vi "errorHandler.vi"(7 "pid":string, 8 "error in":errorcluster, 9 "language":i32, 10 "errNbr":i32, 11 "connection ID":refnum<k5>) -> (0 "error out 2":errorcluster, 3 "connection ID out":refnum<k5>)   [LabVIEW 2016, in "amc_api.lvlib"]
uses:
  amc_api.lvlib
panel:
  out "jsonRespIn":string
  out "JSON-response":string="{\"jsonrpc\":\"2.0\",\"method\":\"\",\"params\":[5,1.245,true,\"name\"],\"id\":\"1\"}"
  out "JSON request":string
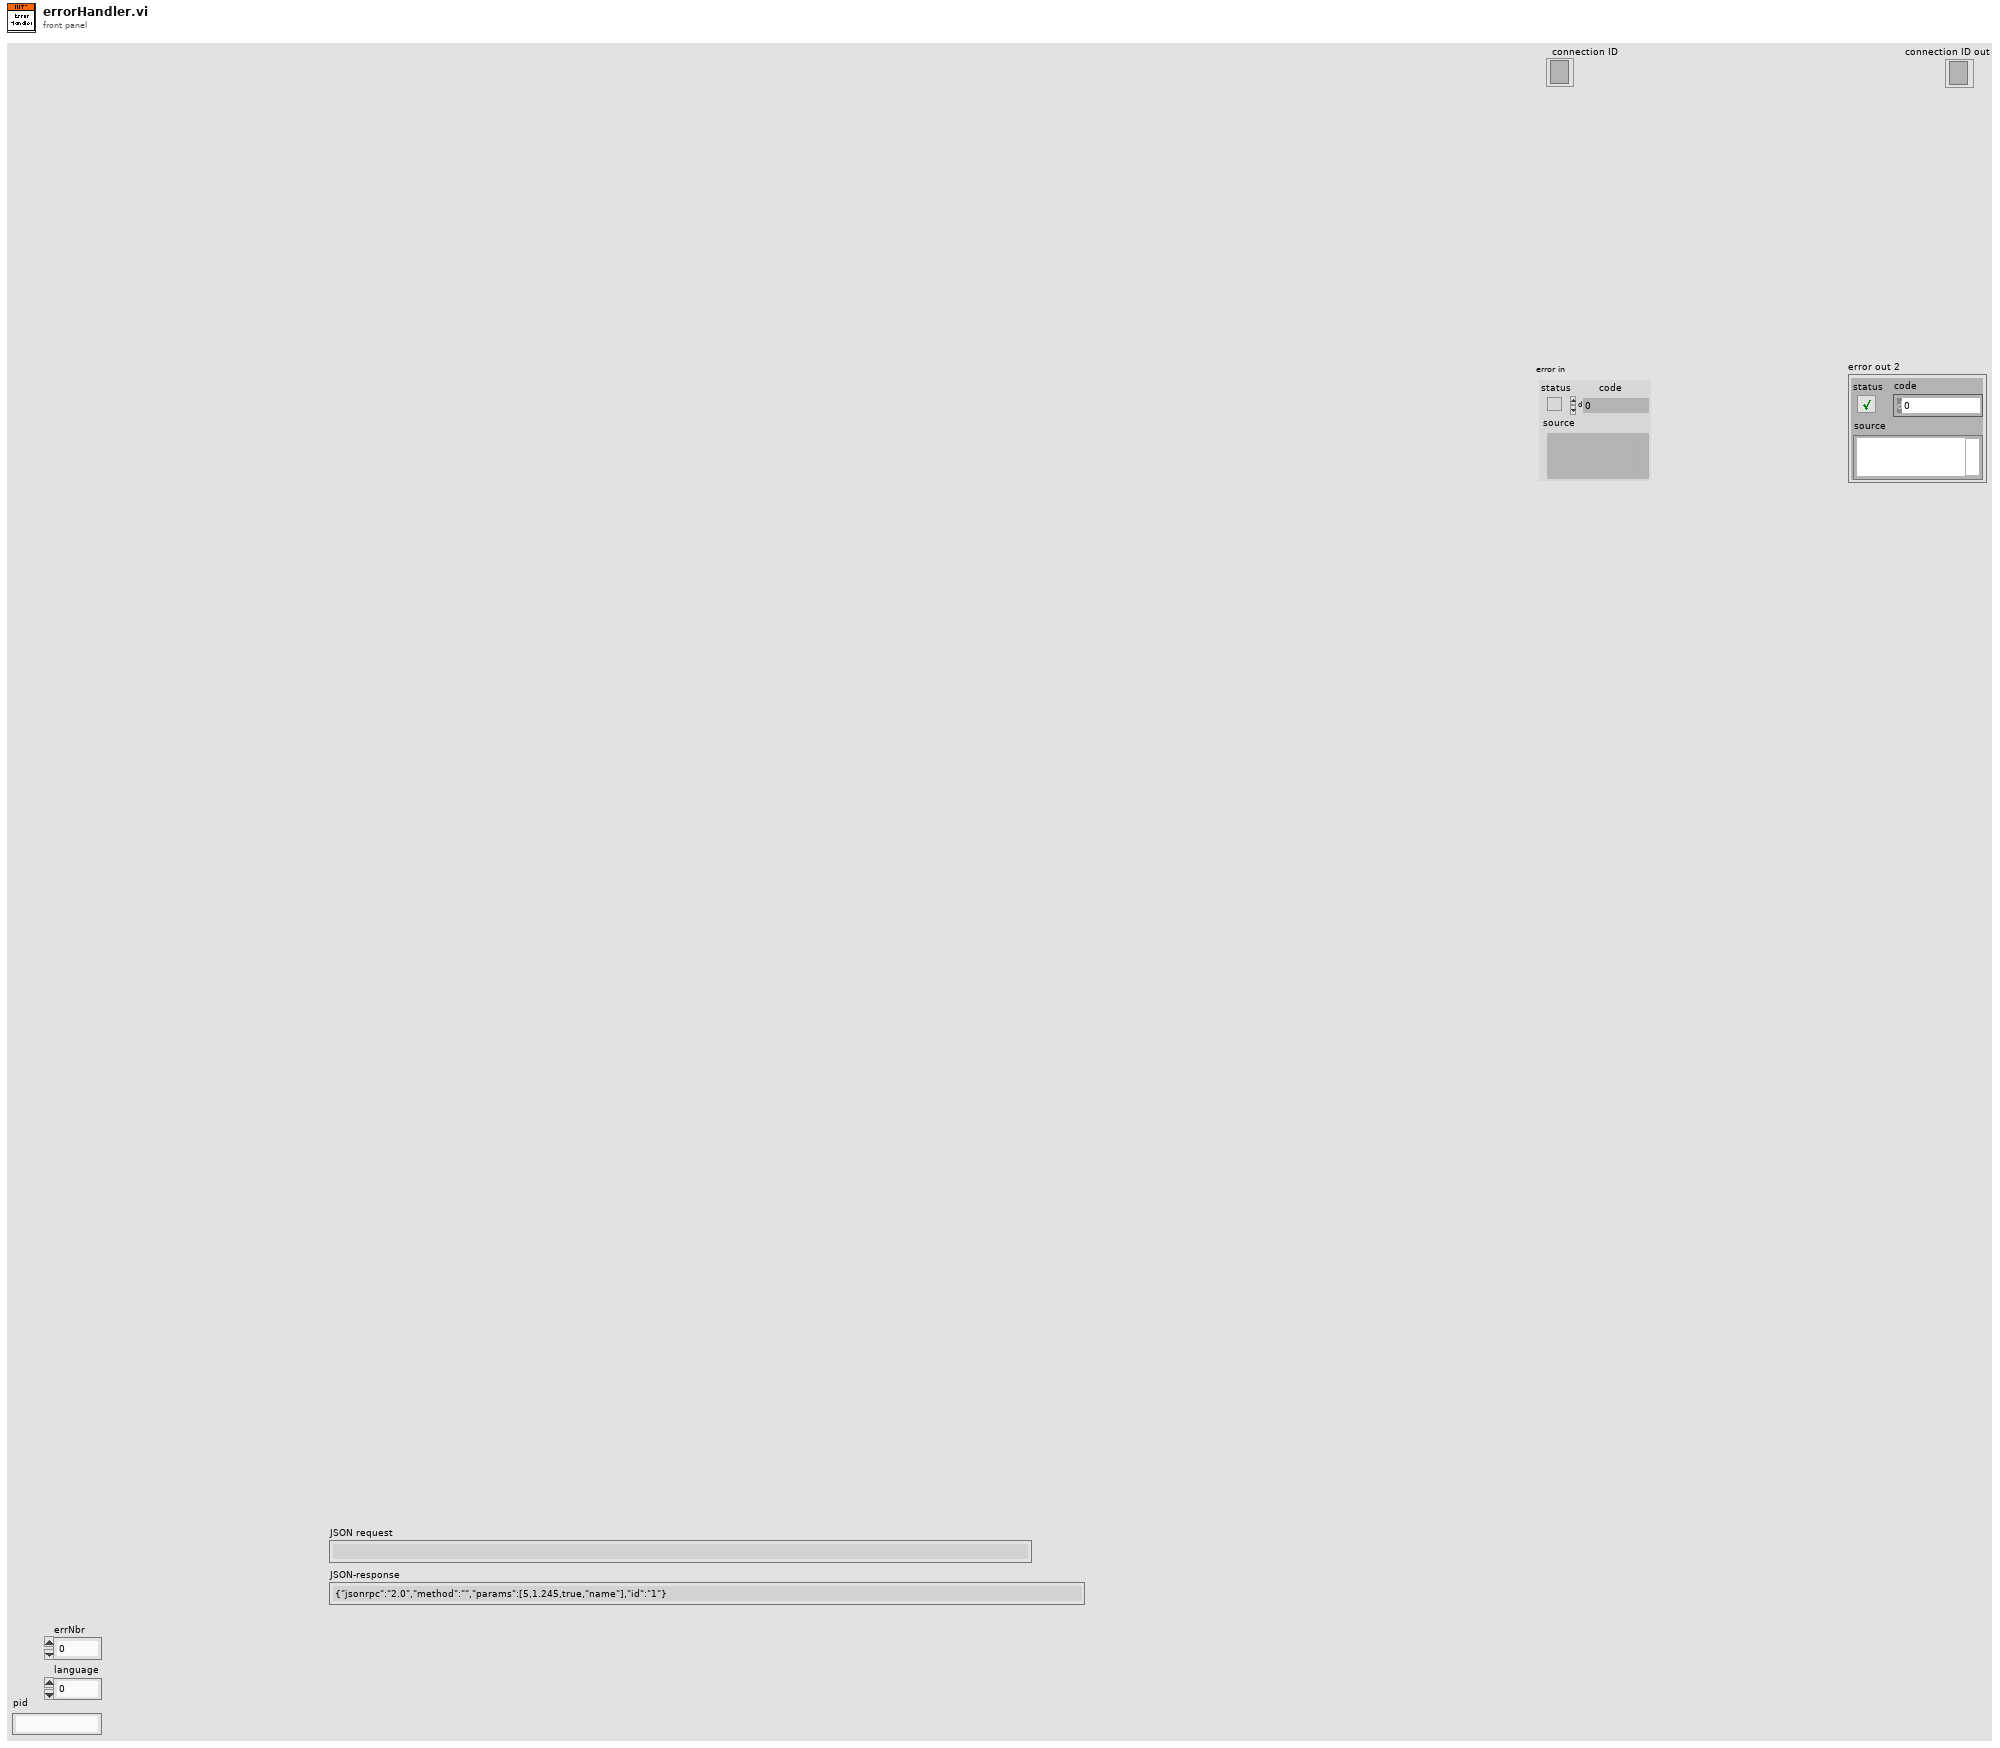
[diagram p1: front panel]
types:
  T1 = cluster{"jsonrpc":string, "method":string, "params":string[], "id":string, "api":i32, "pid":string}
  T2 = enum16{"Standard", "Buffered", "CRLF", "Immediate"}
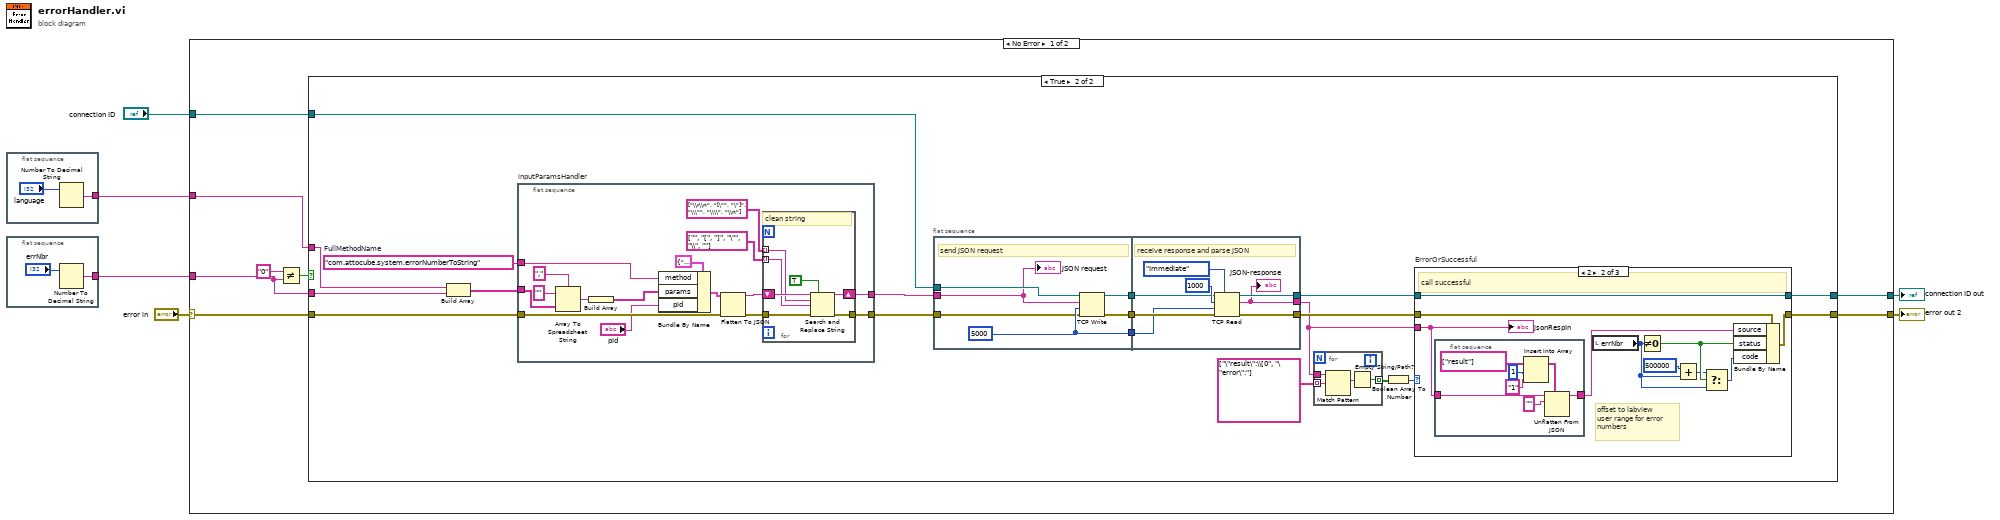
[diagram p0: block diagram]
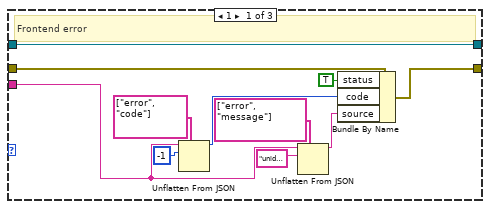
[diagram p3: hidden frame]
diagram:
  n1 = flat-sequence "in_integer" {
    tunnel: [w7] -> w2
    frame #0 {
      n2 = Number To Decimal String(number="language") -> (decimal integer string=w7:string)  [unwired: 1 in]
    }
  }
  n3 = flat-sequence "in_integer" {
    tunnel: [w9] -> w1
    frame #0 {
      n4 = Number To Decimal String(number="errNbr") -> (decimal integer string=w9:string)  [unwired: 1 in]
    }
  }
  n5 = case shown="No Error" "error in" {
    selector: "error in" -> [w14 w112]
    tunnel: [w18 w112] -> w6
    tunnel: [w17 w111] -> w5
    tunnel: "connection ID" -> [w16 w111]
    tunnel: w2 -> [w13 _]
    tunnel: w1 -> [w12 _]
    frame No Error {
      n6 = Not Equal?(x="0", y=w12) -> (x != y?=w15:bool)
      n7 = case shown="True" w15 {
        tunnel: [w20 w30] -> w18
        tunnel: [w19 w29] -> w17
        tunnel: w16 -> [w19 w28]
        tunnel: w12 -> [_ w23]
        tunnel: w14 -> [w20 w24]
        tunnel: w13 -> [_ w22]
        frame False {
        }
        frame True {
          w25 = "com.attocube.system.errorNumberToString"  # FullMethodName
          n8 = Build Array ("ParametersArrayString")(w22, w23) -> (w21:string[])
          n9 = flat-sequence "inputParamsHandler" {
            tunnel: [w43] -> w27
            tunnel: w21 -> [w50]
            tunnel: w24 -> [w48]
            tunnel: [w45] -> w26
            tunnel: w25 -> [w51]
            frame #0 {
              n10 = Array To Spreadsheet String(delimiter (Tab)=",", array=w50, 3:"" ("format string")) -> (spreadsheet string=w53:string)
              n11 = Build Array "Build Array"(w53) -> (w49:string[])
              n12 = Bundle By Name(cluster=T1 {"jsonrpc"="2.0", "method"="com.attocube.amc.res.setRESReadOutFreq", "params"=[], "id"="1", "api"=2, "pid"=""}, "method"=w51, "params"=w49, "pid"="pid") -> (w52:T1)
              n13 = Flatten To JSON(anything=w52, error in (no error)=w48) -> (JSON string=w44:string, 11:w46:errorcluster)  [unwired: 1 in]
              n14 = for {
                tunnel: string[] ["\\r\\n", "[\"", "\"]", "\\\"", "\\\\", "\\n"] ("search string") -> [w59] mode=indexing
                tunnel: string[] ["", "[", "]", "\"", "\\", ""] ("replace string (\"\")") -> [w58] mode=indexing
                shift-right: [w61] -> w43
                shift-left: w44 -> [w60]
                tunnel: w46 -> [w57]
                tunnel: [w56] -> w45
                # "clean string"
                n15 = Search and Replace String(replace all?=TRUE ("replace all? (F)"), input string=w60, search string=w59, replace string=w58, error in=w57) -> (result string=w61:string, error out=w56:errorcluster)  [unwired: 3 in, 2 out]
              }
            }
          }
          n16 = flat-sequence {
            tunnel: w28 -> [w102]
            tunnel: [w100] -> w39
            tunnel: [w101] -> w38
            tunnel: w26 -> [w97]
            tunnel: [w99] -> w37
            tunnel: w27 -> [w98]
            tunnel: [w106] -> w33
            tunnel: w39 -> [w108]
            tunnel: w38 -> [w107]
            tunnel: [w104] -> w32
            tunnel: w37 -> [w105]
            tunnel: [w103] -> w31
            frame #0 {
              w99 = 5000 ("timeout ms (25000)")
              # "send JSON request"
              n17 = TCP Write(connection ID=w102, data in=w98, error in (no error)=w97, 9:w99) -> (connection ID out=w100:refnum<k5>, error out=w101:errorcluster)  [unwired: 1 out]
              "JSON request" <- w98
            }
            frame #1 {
              # "receive response and parse JSON"
              n18 = TCP Read(connection ID=w108, bytes to read=1000, error in (no error)=w107, 7:T2."Immediate" ("mode (standard)"), 9:w105) -> (connection ID out=w106:refnum<k5>, data out=w103:string, error out=w104:errorcluster)
              "JSON-response" <- w103
            }
          }
          n19 = for {
            tunnel: string[] ["\"result\":\\[0", "\"error\":"] ("path") -> [w65] mode=indexing
            tunnel: [w63] -> w35 mode=indexing
            tunnel: w31 -> [w66]
            n20 = Match Pattern(string=w66, regular expression=w65) -> (match substring=w64:string)  [unwired: 1 in, 3 out]
            n21 = Empty String/Path?(string/path=w64) -> (empty?=w63:bool)
          }
          n22 = Boolean Array To Number(Boolean array=w35) -> (number=w34:u32)
          n23 = case "ErrorOrSuccessful" shown="2" w34 {
            tunnel: w31 -> [w69 w84 _]
            tunnel: w33 -> [w70 w87 w96]
            tunnel: [w70 w87 w96] -> w29
            tunnel: [w71 w85 w95] -> w30
            tunnel: w32 -> [w72 w86 w95]
            frame 1 {
              # "Frontend error"
              n24 = Unflatten From JSON(path=string[] ["error", "code"], JSON string=w69, type and defaults=-1) -> (value=w74:i32)  [unwired: 4 in, 1 out]
              n25 = Unflatten From JSON(path=string[] ["error", "message"], JSON string=w69, type and defaults="unidentified error") -> (value=w73:string)  [unwired: 4 in, 1 out]
              n26 = Bundle By Name(cluster=w72, "status"=TRUE, "code"=w74, "source"=w73) -> (w71:errorcluster)
            }
            frame 2 {
              # "offset to labview\nuser range for error\nnumbers"
              # "call successful"
              n27 = flat-sequence "out_string" {
                tunnel: w84 -> [w94]
                tunnel: [w88] -> w83
                frame #0 {
                  n28 = Insert Into Array(array=string[] ["result"] ("path"), index=1, new element="1" ("idx")) -> (w91:string[])
                  n29 = Unflatten From JSON(path=w91, JSON string=w94, type and defaults="") -> (value=w88:string)  [unwired: 4 in, 1 out]
                }
              }
              n30 = local read "errNbr"() -> (w78:i32)
              n31 = Not Equal To 0?(x=w78) -> (x != 0?=w81:bool)
              n32 = Add(x=500000 ("y"), y=w78) -> (x+y=w80:i32)
              n33 = Select(t=w80, s=w81, f=w78) -> (s? t:f=w82:i32)
              n34 = Bundle By Name(cluster=w86, "source"=w83, "status"=w81, "code"=w82) -> (w85:errorcluster)
              "jsonRespIn" <- w84
            }
            frame Default {
            }
          }
        }
      }
    }
    frame Error {
    }
  }
  "error out 2" <- w6
  "connection ID out" <- w5
